vi "Read Card #.vi"(8 "error in (no error)":errorcluster, 11 "Generic Card in":refnum<class "Generic Card.lvclass">) -> (0 "error out":errorcluster, 2 "Card #":dbl, 3 "Generic Card out":refnum<class "Generic Card.lvclass">)   [LabVIEW 2012, in "Generic Instrument.lvlib" / "Generic Card.lvclass"]
uses:
  Generic Card.lvclass
  Generic Card.lvclass/Generic Card.ctl
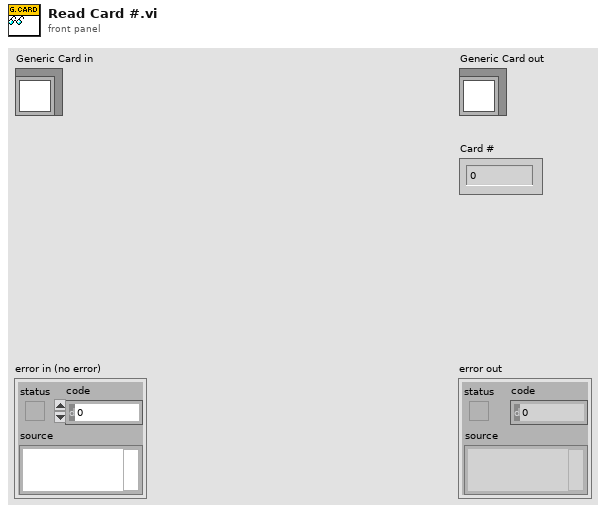
[diagram p1: front panel]
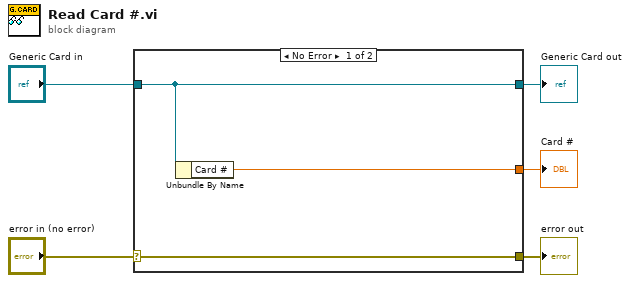
[diagram p0: block diagram]
diagram:
  n1 = case shown="No Error" "error in (no error)" {
    selector: "error in (no error)" -> [w8 w9]
    tunnel: [w8 w9] -> w4
    tunnel: [w7 w10] -> w2
    tunnel: "Generic Card in" -> [w7 w10]
    tunnel: [w6 _] -> w1
    frame No Error {
      n2 = Unbundle By Name(w7) -> ("Card #"=w6:dbl)
    }
    frame Error {
    }
  }
  "error out" <- w4
  "Generic Card out" <- w2
  "Card #" <- w1
